vi "Get String Message.vi"(8 "error in (no error)":errorcluster, 11 "Message String in":refnum<class "Message String.lvclass">) -> (0 "error out":errorcluster, 1 "Value":string, 2 "Name":string, 3 "Message String out":refnum<class "Message String.lvclass">)   [LabVIEW 2016, in "Stream Mediator.lvlib" / "Message String.lvclass"]
doc: "--\nCopyright © 2017 Composed SystemsI All rights reserved.\n\nAuthor: Jon McBee <jon.mcbee@composed.io>\n\nThis library is provided \"AS IS\" ,WITHOUT WARRANTIES OR\nCONDITIONS OF ANY KIND, either express or implied.\n\nComposed Systems -- composed.io\n\nStream 0.0.1.1\nJon McBee - Composed Systems\nCopyright (c) 2017, Composed Systems"
uses:
  <userlib>/Composed Systems/Stream/Mediator/Classes/Message String/Message String.lvclass
  C:/Program Files (x86)/National Instruments/LabVIEW 2016/user.lib/Composed Systems/Stream/Mediator/Classes/Message Interface/Message Interface.lvclass
  <userlib>/Composed Systems/Stream/Mediator/Classes/Message String/Message String.lvclass/Message String.ctl
  <userlib>/Composed Systems/Stream/Mediator/Classes/Message Interface/Message Interface.lvclass
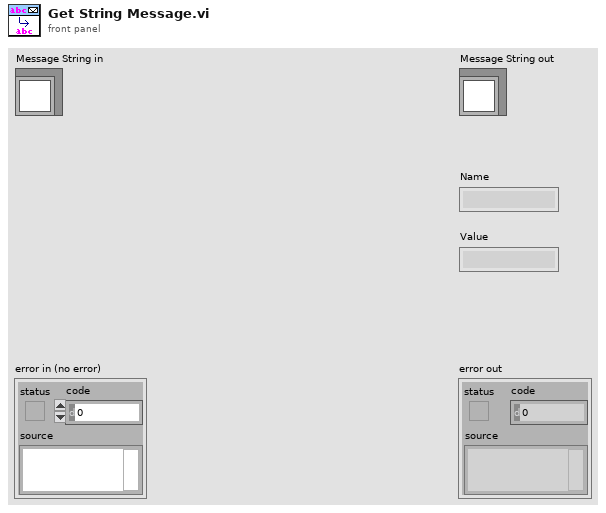
[diagram p1: front panel]
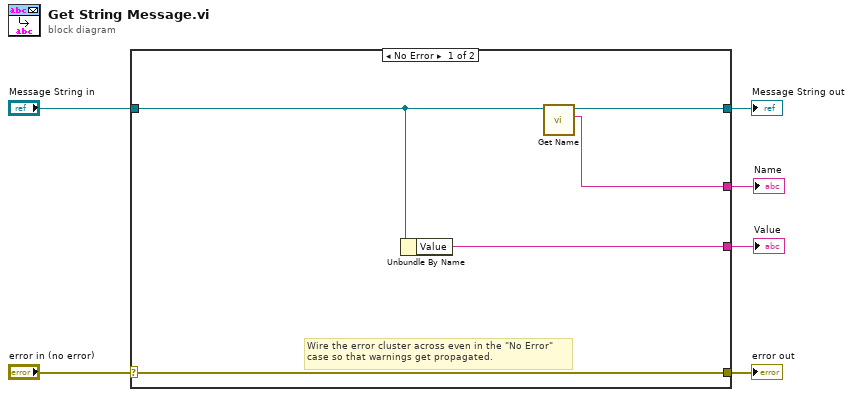
[diagram p0: block diagram]
diagram:
  n1 = case shown="No Error" "error in (no error)" {
    selector: "error in (no error)" -> [w11 w13]
    tunnel: [w11 w13] -> w5
    tunnel: [w8 w12] -> w3
    tunnel: "Message String in" -> [w9 w12]
    tunnel: [w10 _] -> w2
    tunnel: [w7 _] -> w1
    frame No Error {
      # "Wire the error cluster across even in the \"No Error\"\ncase so that warnings get propagated."
      n2 = Unbundle By Name(w9) -> ("Value"=w10:string)
      n3 = call <userlib>:"Get Name.vi"("Message Interface in"=w9) -> ("Name"=w7:string, "Message Interface out"=w8:refnum<class "Message String.lvclass">)  [unwired: 8 in, 1 out]
    }
    frame Error {
    }
  }
  "error out" <- w5
  "Message String out" <- w3
  "Name" <- w1
  "Value" <- w2
